vi "Add New Tower.vi"(3 "Main Scene Object Ref":refnum<vi>, 5 "Tower Height":sgl, 6 "Indices":i32[](array[numeric]), 7 "3D Scene reference":refnum<vi>, 8 "Voronoi Y vertices":dbl[](array[numeric]), 9 "Voronoi X vertices":dbl[](array[numeric]), 10 "Location":T1, 11 "Voronoi grid ref":refnum<vi>) -> (0 "error out":errorcluster)   [LabVIEW 2023]
doc: "Add a new tower to the 3D Picture."
uses:
  <vilib>/Utility/miscctls.llb/LV3DPointTypeDef.ctl
  <vilib>/Utility/miscctls.llb/LVRGBAColorTypeDef.ctl
  <vilib>/picture/3D Picture Control/Object/Add Object (reference).vi
  <vilib>/picture/3D Picture Control/NI_3D Picture Control.lvlib
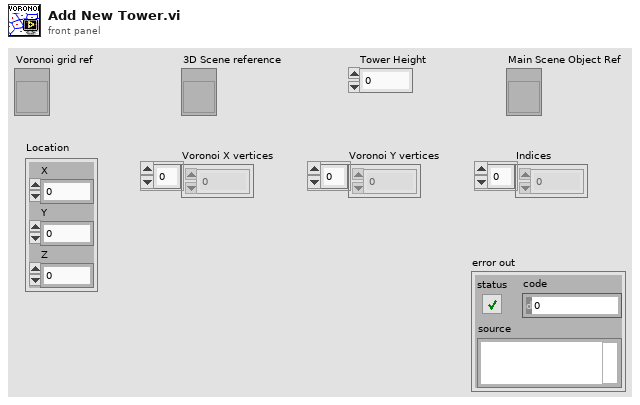
[diagram p1: front panel]
types:
  T1 = typedef "LV3DPointTypeDef.ctl" = cluster{"X":sgl, "Y":sgl, "Z":sgl}
  T2 = typedef "LVRGBAColorTypeDef.ctl" = cluster{"Red":sgl, "Green":sgl, "Blue":sgl, "Alpha":sgl}
  T3 = enum16{"Overall", "Per Primitive", "Per Vertex", "Binding Off"}
  T4 = enum16{"Points", "Lines", "Line Strip", "Line Loop", "Triangles", "Triangle Strip", "Triangle Fan", "Quads", "Quad Strip", "Polygon"}
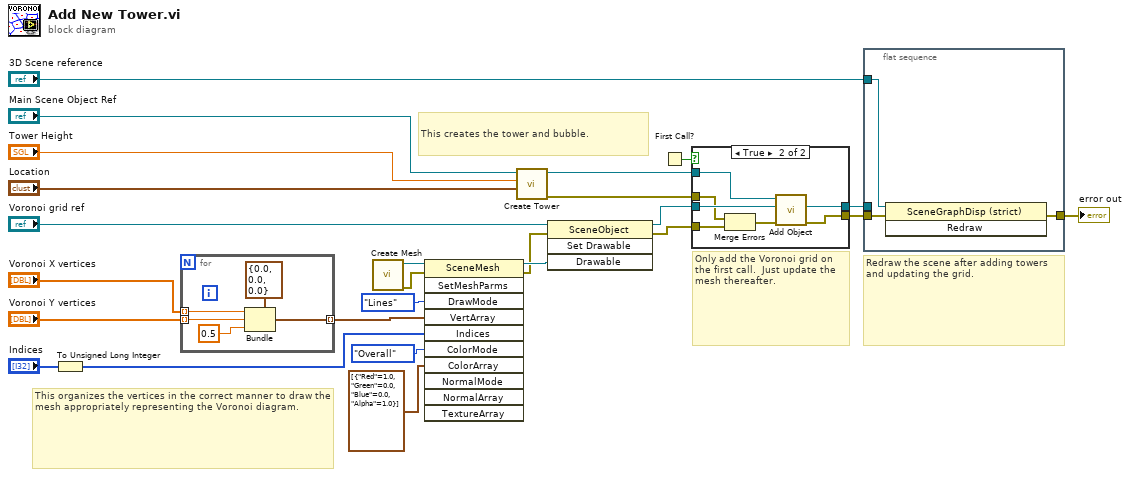
[diagram p0: block diagram]
diagram:
  # "Redraw the scene after adding towers and updating the grid."
  # "Only add the Voronoi grid on the first call.  Just update the mesh thereafter."
  # "This creates the tower and bubble."
  # "This organizes the vertices in the correct manner to draw the mesh appropriately representing the Voronoi diagram."
  n1 = To Unsigned Long Integer(number="Indices") -> (unsigned 32bit integer=w11:u32[])
  n2 = for {
    tunnel: "Voronoi X vertices" -> [w29] mode=indexing
    tunnel: "Voronoi Y vertices" -> [w28] mode=indexing
    tunnel: [w27] -> w1 mode=indexing
    n3 = Bundle(cluster=T1 {"X"=0.0, "Y"=0.0, "Z"=0.0} ("3D Point"), "X"=w29, "Y"=w28, "Z"=sgl 0.5) -> (w27:T1)
  }
  n4 = call <vilib>:"Create Mesh.vi"() -> ("error out"=w7:errorcluster, "New Mesh Refnum"=w21:refnum<vi>)  [unwired: 1 in, 9 out]
  n5 = invoke class="SceneMesh" method="SetMeshParms"(reference=w21, error in=w7, "DrawMode"=T4."Lines" ("Draw Mode"), "VertArray"=w1, "Indices"=w11, "ColorMode"=T3."Overall" ("Color Binding Mode"), "ColorArray"=T2[] [{"Red"=1.0, "Green"=0.0, "Blue"=0.0, "Alpha"=1.0}] ("Color Array")) -> (reference out=w20:refnum<vi>, error out=w6:errorcluster)  [unwired: 4 in, 9 out]
  n6 = call "Create Tower.vi"("Location"="Location", "Tower Height"="Tower Height", "Main Scene Object"="Main Scene Object Ref") -> ("error out"=w3:errorcluster, "Main Scene Object (out)"=w16:refnum<vi>)  [unwired: 1 in, 6 out]
  n7 = invoke class="SceneObject" method="Set Drawable"(reference="Voronoi grid ref", error in=w6, "Drawable"=w20) -> (reference out=w25:refnum<vi>, error out=w4:errorcluster)  [unwired: 1 in, 2 out]
  n8 = First Call?() -> (First Call?: T/F=w10:bool)
  n9 = case shown="True" w10 {
    tunnel: w25 -> [w32 w38]
    tunnel: [w32 w33] -> w9
    tunnel: w16 -> [_ w39]
    tunnel: [w31 w37] -> w5
    tunnel: w4 -> [w31 w36]
    tunnel: w3 -> [_ w35]
    frame False {
    }
    frame True {
      n10 = Merge Errors(w35, w36) -> (w34:errorcluster)
      n11 = call-poly <vilib>:"Add Object.vi"("error in (no error)"=w34, "New Object In"=w38, "Scene Object In"=w39) -> ("error out"=w37:errorcluster, "New Object Out"=w33:refnum<vi>)  [unwired: 6 in, 1 out]
    }
  }
  n12 = flat-sequence {
    tunnel: w9 -> [_]
    tunnel: "3D Scene reference" -> [w42]
    tunnel: w5 -> [w41]
    tunnel: [w40] -> w2
    frame #0 {
      n13 = invoke class="SceneGraphDisp (strict)" method="Redraw"(reference=w42, error in=w41) -> (error out=w40:errorcluster)  [unwired: 1 in, 2 out]
    }
  }
  "error out" <- w2
